vi "ConvertVoltageToFrequency.vi"(9 "PSU":string, 10 "Charging Voltage [kV]":dbl, 11 "Calibration Folderpath":path) -> (3 "Frequency [Hz]":dbl)   [LabVIEW 2014]
uses:
  <vilib>/Utility/file.llb/Read From Spreadsheet File (DBL).vi
  <vilib>/gmath/NI_Gmath.lvlib
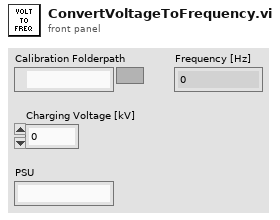
[diagram p1: front panel]
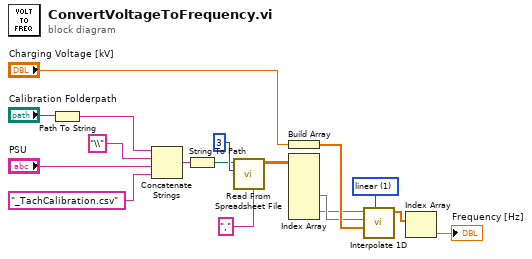
[diagram p0: block diagram]
diagram:
  w15 = 1 items=["nearest", "linear", "spline", "cubic Hermite", "Lagrange"] ("method")
  n1 = Path To String(path="Calibration Folderpath") -> (string=w3:string)
  n2 = Concatenate Strings(w3, "\\" ("string"), "PSU", "_TachCalibration.csv" ("string")) -> (w7:string)
  n3 = String To Path(string=w7) -> (path=w8:path)
  n4 = call-poly <vilib>:"Read From Spreadsheet File.vi"("delimiter (\\t)"="," ("delimiter (\\t)"), "number of rows (all:-1)"=3, "file path (dialog if empty)"=w8) -> ("all rows"=w11:dbl[][])  [unwired: 4 in, 4 out]
  n5 = Build Array("Charging Voltage [kV]") -> (w14:dbl[])
  n6 = Index Array(array=w11) -> (element #2=w13:dbl[], element #3=w12:dbl[])  [unwired: 6 in, 1 out]
  n7 = call <vilib>:"Interpolate 1D.vi"("method"=w15, "xi"=w14, "X"=w13, "Y"=w12) -> ("yi"=w16:dbl[])  [unwired: 5 in, 2 out]
  n8 = Index Array(array=w16) -> (element=→"Frequency [Hz]":dbl)  [unwired: 1 in]
